vi "Main_GOOP4_CreateObjects_Open_GDS.vi"() -> ()   [LabVIEW 2019]
doc: "This is the main VI for the Project \"GOOP4_CreateObjects_Open_GDS.lvproj\""
uses:
  GOOP4_Sub_class/GOOP4_Sub.lvclass
  GOOP4_Base_class/GOOP4_Base.lvclass
panel:
  out "Sub Str":string
  out "Sub error out":errorcluster
  out "Base error out":errorcluster
  out "Sub i 1":i32
  out "Sub i 2":i32
  out "Base i 2":i32
  out "Base i 1":i32
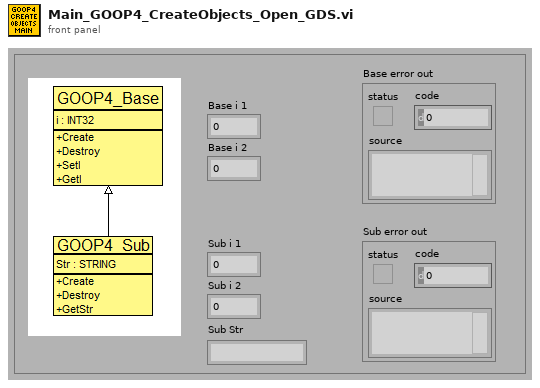
[diagram p1: front panel]
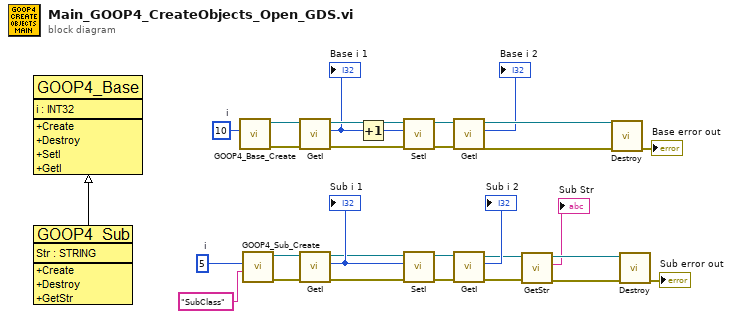
[diagram p0: block diagram]
diagram:
  w17 = 5  # i
  w25 = 10  # i
  n1 = call "GOOP4_Base_Create.vi"("i"=w25) -> ("error out"=w23:errorcluster, "reference out"=w24:refnum<class "GOOP4_Base.lvclass">)  [unwired: 9 in]
  n2 = call "GOOP4_Sub_Create.vi"("Str"="SubClass", "i"=w17) -> ("error out"=w9:errorcluster, "reference out"=w8:refnum<class "GOOP4_Sub.lvclass">)  [unwired: 8 in]
  n3 = call-dynamic "GetI.vi"("error in (no error)"=w23, "reference in"=w24) -> ("error out"=w21:errorcluster, "i"=w20:i32, "reference out"=w22:refnum<class "GOOP4_Base.lvclass">)  [unwired: 7 in]
  "Base i 1" <- w20
  n4 = call-dynamic "GetI.vi"("error in (no error)"=w9, "reference in"=w8) -> ("error out"=w13:errorcluster, "i"=w14:i32, "reference out"=w12:refnum<class "GOOP4_Sub.lvclass">)  [unwired: 7 in]
  "Sub i 1" <- w14
  n5 = Increment(x=w20) -> (x+1=w19:i32)
  n6 = call-dynamic "SetI.vi"("error in (no error)"=w21, "i"=w19, "reference in"=w22) -> ("error out"=w29:errorcluster, "reference out"=w28:refnum<class "GOOP4_Base.lvclass">)  [unwired: 7 in]
  n7 = call-dynamic "SetI.vi"("error in (no error)"=w13, "i"=w14, "reference in"=w12) -> ("error out"=w10:errorcluster, "reference in"=w11:refnum<class "GOOP4_Sub.lvclass">)  [unwired: 7 in]
  n8 = call-dynamic "GetI.vi"("error in (no error)"=w29, "reference in"=w28) -> ("error out"=w26:errorcluster, "i"=→"Base i 2":i32, "reference out"=w27:refnum<class "GOOP4_Base.lvclass">)  [unwired: 7 in]
  n9 = call-dynamic "GetI.vi"("error in (no error)"=w10, "reference in"=w11) -> ("error out"=w6:errorcluster, "i"=→"Sub i 2":i32, "reference out"=w7:refnum<class "GOOP4_Sub.lvclass">)  [unwired: 7 in]
  n10 = call-dynamic "GetStr.vi"("error in (no error)"=w6, "reference in"=w7) -> ("error out"=w4:errorcluster, "Str"=→"Sub Str":string, "reference in"=w5:refnum<class "GOOP4_Sub.lvclass">)  [unwired: 7 in]
  n11 = call-dynamic "Destroy.vi"("error in (no error)"=w26, "reference in"=w27) -> ("error out"=→"Base error out":errorcluster)  [unwired: 8 in, 1 out]
  n12 = call-dynamic "Destroy.vi"("error in (no error)"=w4, "reference in"=w5) -> ("error out"=→"Sub error out":errorcluster)  [unwired: 8 in, 1 out]
